vi "Setup DIO64 for Output.vi"(0 "timestamps (ms)":dbl[](array[numeric]) format="%.3f", 1 "scan rate (Hz)":dbl=5000000.0 format="%.2f", 5 "bitmap":bool[][](array[boolean]), 7 "output cluster":cluster{bool[][], bool[][], bool[][], bool[][]}) -> (10 "data":u16[][](array[numeric])=[[1]] format="%.0x")   [LabVIEW 2012]
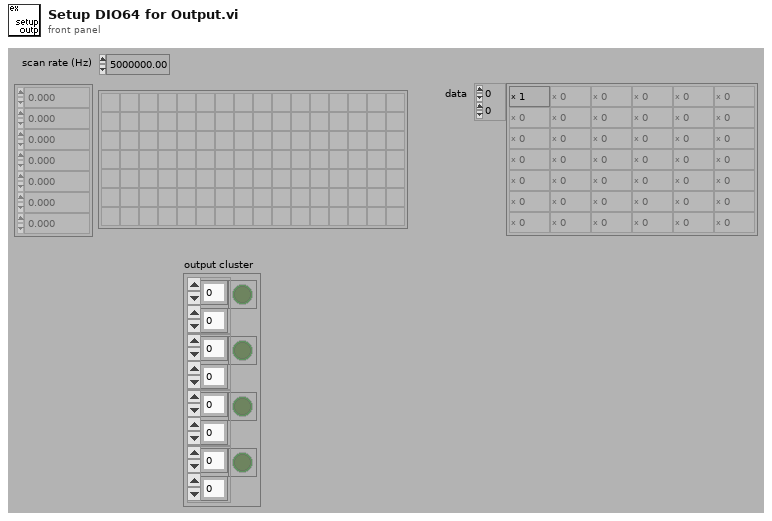
[diagram p1: front panel]
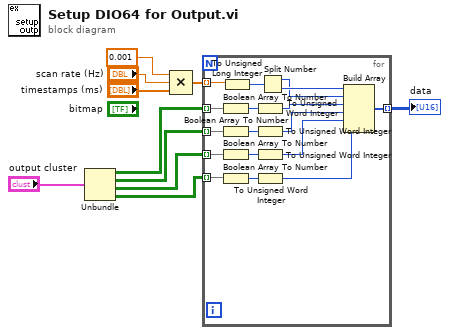
[diagram p0: block diagram]
diagram:
  n1 = Unbundle("output cluster") -> (w4:bool[][], w3:bool[][], w2:bool[][], w1:bool[][])
  n2 = Compound Arithmetic op=MULTIPLY(0.001 ("x"), "scan rate (Hz)", "timestamps (ms)") -> (w6:dbl[])
  n3 = for {
    tunnel: w6 -> [w21] mode=indexing
    tunnel: w4 -> [w27] mode=indexing
    tunnel: [w22] -> w10 mode=indexing
    tunnel: w3 -> [w15] mode=indexing
    tunnel: w2 -> [w14] mode=indexing
    tunnel: w1 -> [w13] mode=indexing
    n4 = Boolean Array To Number(Boolean array=w27) -> (number=w26:u32)
    n5 = Boolean Array To Number(Boolean array=w15) -> (number=w19:u32)
    n6 = Boolean Array To Number(Boolean array=w14) -> (number=w17:u32)
    n7 = Boolean Array To Number(Boolean array=w13) -> (number=w16:u32)
    n8 = To Unsigned Long Integer(number=w21) -> (unsigned 32bit integer=w25:u32)
    n9 = To Unsigned Word Integer(number=w26) -> (unsigned 16bit integer=w20:u16)
    n10 = To Unsigned Word Integer(number=w19) -> (unsigned 16bit integer=w18:u16)
    n11 = To Unsigned Word Integer(number=w17) -> (unsigned 16bit integer=w12:u16)
    n12 = To Unsigned Word Integer(number=w16) -> (unsigned 16bit integer=w11:u16)
    n13 = Split Number(x=w25) -> (hi(x)=w23:u16, lo(x)=w24:u16)
    n14 = Build Array(w24, w23, w20, w18, w12, w11) -> (w22:u16[])
  }
  "data" <- w10
